vi "moveToPosition.vi"(6 "Delay between send and receive [ms]":i32=100, 8 "error in (no error)":errorcluster, 10 "wavelength":dbl format="%#_13g", 11 "Monochromator in":refnum<class "Monochromator.lvclass">) -> (0 "error out":errorcluster, 1 "ID":i32, 2 "results-JSON string":string, 3 "Monochromator out":refnum<class "Monochromator.lvclass">)   [LabVIEW 2020, in "horiba.lvlib" / "Monochromator.lvclass"]
doc: "This command starts the monochromator moving to the requested wavelength in nm. This is an asynchronous command. Use the mono_isBusy command to know when the move has completed."
uses:
  Monochromator.lvclass
  Monochromator.lvclass/Monochromator.ctl
  7fe8abea-6ecd-46de-aa11-ce8637911b6a.vi
  GenericDevice/GenericDevice.lvclass
  35d46a5a-fd7c-4445-96f4-e877dae8f93b.vi
panel:
  # "Connector Pane"
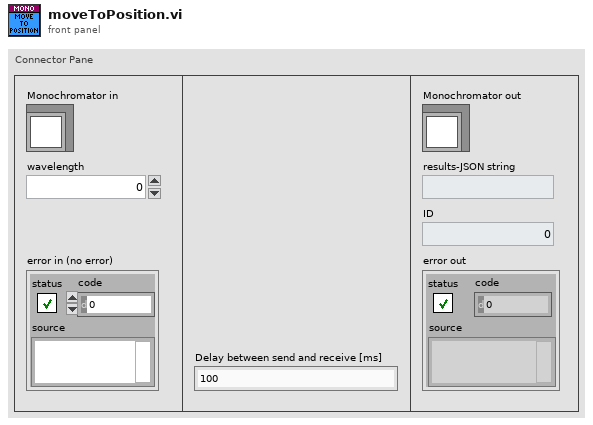
[diagram p1: front panel]
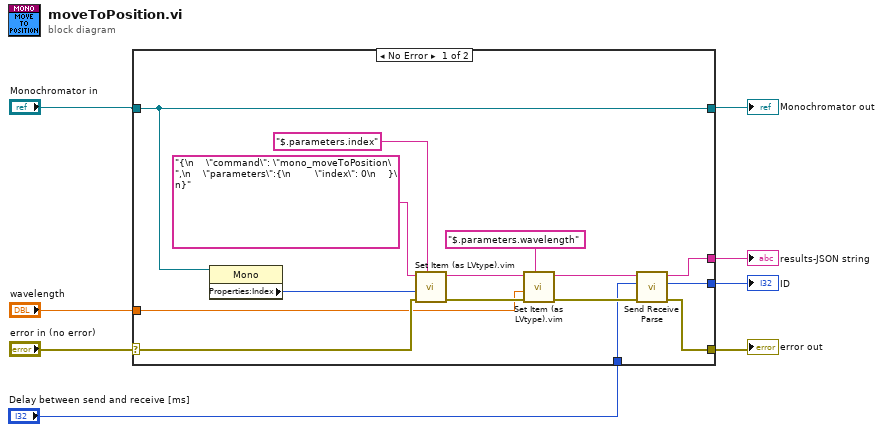
[diagram p0: block diagram]
diagram:
  n1 = case shown="No Error" "error in (no error)" {
    selector: "error in (no error)" -> [w19 w25]
    tunnel: [w16 w25] -> w5
    tunnel: [w21 w24] -> w7
    tunnel: "Monochromator in" -> [w21 w24]
    tunnel: [w18 _] -> w3
    tunnel: [w17 _] -> w4
    tunnel: "wavelength" -> [w10 _]
    tunnel: "Delay between send and receive [ms]" -> [w9 _]
    frame No Error {
      n2 = property class="Mono"(reference=w21) -> ("Properties:Index"=w20:i32)  [unwired: 1 in, 2 out]
      n3 = call "Set Item (as LVtype).vim"("$Path or Item Name"="$.parameters.index", "error in (no error)"=w19, "Anything"=w20, "JSON"="{\n    \"command\": \"mono_moveToPosition\",\n    \"parameters\":{\n        \"index\": 0\n    }\n}") -> ("error out"=w14:errorcluster, "<JSON>"=w12:string)  [unwired: 4 in, 1 out]
      n4 = call "Set Item (as LVtype).vim"("$Path or Item Name"="$.parameters.wavelength", "error in (no error)"=w14, "Anything"=w10, "JSON"=w12) -> ("error out"=w13:errorcluster, "<JSON>"=w11:string)  [unwired: 4 in, 1 out]
      n5 = call "Send Receive Parse.vi"("error in"=w13, "Delay between send and receive [ms]"=w9, "<JSON>"=w11) -> ("error out"=w16:errorcluster, "ID"=w17:i32, "results-JSON string"=w18:string)  [unwired: 6 in]
    }
    frame Error {
    }
  }
  "error out" <- w5
  "Monochromator out" <- w7
  "ID" <- w4
  "results-JSON string" <- w3
